vi "Set Slave Info.vi"(8 "error in (no error)":errorcluster, 10 "Slave Info":T1, 11 "Master Device in":refnum<class "Master Device.lvclass">) -> (0 "error out":errorcluster, 3 "Master Device out":refnum<class "Master Device.lvclass">)   [LabVIEW 2013, in "Master Device.lvclass"]
uses:
  Master Device.lvclass
  TypeDefs/SlaveInfo.ctl
  TypeDefs/RampInfo.ctl
  Master Device.lvclass/Master Device.ctl
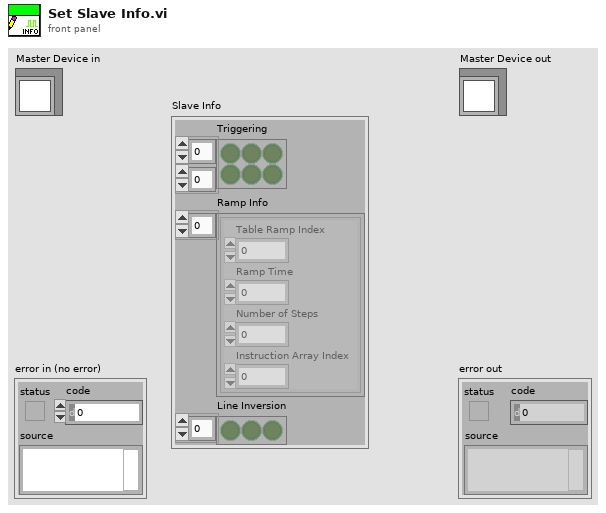
[diagram p1: front panel]
types:
  T1 = typedef "SlaveInfo.ctl" = cluster{"Triggering":bool[][], "Ramp Info":T2[], "Line Inversion":bool[]}
  T2 = typedef "RampInfo.ctl" = cluster{"Table Ramp Index":i32, "Ramp Time":dbl, "Number of Steps":i32, "Instruction Array Index":i32}
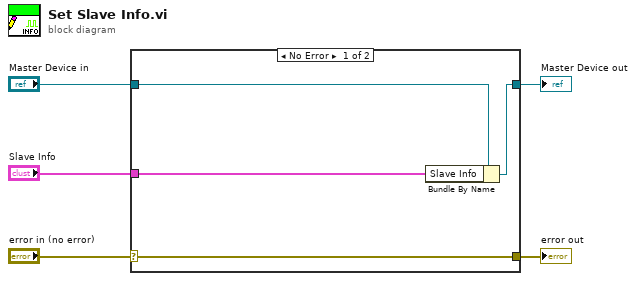
[diagram p0: block diagram]
diagram:
  n1 = case shown="No Error" "error in (no error)" {
    selector: "error in (no error)" -> [w9 w10]
    tunnel: [w9 w10] -> w4
    tunnel: [w7 w11] -> w2
    tunnel: "Master Device in" -> [w8 w11]
    tunnel: "Slave Info" -> [w6 _]
    frame No Error {
      n2 = Bundle By Name(cluster=w8, "Slave Info"=w6) -> (w7:refnum<class "Master Device.lvclass">)
    }
    frame Error {
    }
  }
  "error out" <- w4
  "Master Device out" <- w2
